vi "Actor Core.vi"(8 "error in":errorcluster, 11 "Progress Window in":refnum<class "Progress Window.lvclass">) -> (0 "error out":errorcluster, 3 "Actor out":refnum<class "Actor.lvclass">)   [LabVIEW 2018, in "Progress Window.lvlib" / "Progress Window.lvclass"]
doc: "(<B>Filename</B>: Actor Framework.lvlib:Actor.lvclass:Actor Core.vi)\n\nReceives messages to the actor, reacts to them, and initiates any error handling that may shut the actor down.\n\nDescendant classes may override this VI to append parallel tasks for the actor to complete while it handles messages. Overrides use the Call Parent Method node."
uses:
  Progress Window.lvclass
  C:/Program Files/National Instruments/LabVIEW 2018/vi.lib/ActorFramework/Actor/Actor.lvclass
  C:/LVCUR/flash-gordon/User Interface/UI Window/UI Window.lvclass
  <vilib>/ActorFramework/Actor/Actor.lvclass
  <vilib>/ActorFramework/Actor/Actor.lvclass/Actor.ctl
  <vilib>/ActorFramework/Message Enqueuer/Message Enqueuer.lvclass/Message Enqueuer.ctl
  <vilib>/ActorFramework/Message Enqueuer/Init from Existing Queue.vi
  <vilib>/ActorFramework/Message Enqueuer/Enqueue.vi
  <vilib>/ActorFramework/Stop Msg/Stop Msg.lvclass
  C:/Program Files/National Instruments/LabVIEW 2018/vi.lib/ActorFramework/Message/Message.lvclass
  Resources/GLOBAL/GLOBAL Time-critical.vi
  <vilib>/ActorFramework/Message Priority Queue/Priority Enqueue.vi
  UI Window/UI Window.lvclass
  <vilib>/ActorFramework/Message Enqueuer/Message Enqueuer.lvclass
panel:
  in  "Stop Button":bool
  out "Recording Movie":u8(slide) scale=0.0..100.0
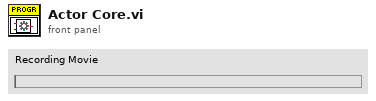
[diagram p1: front panel]
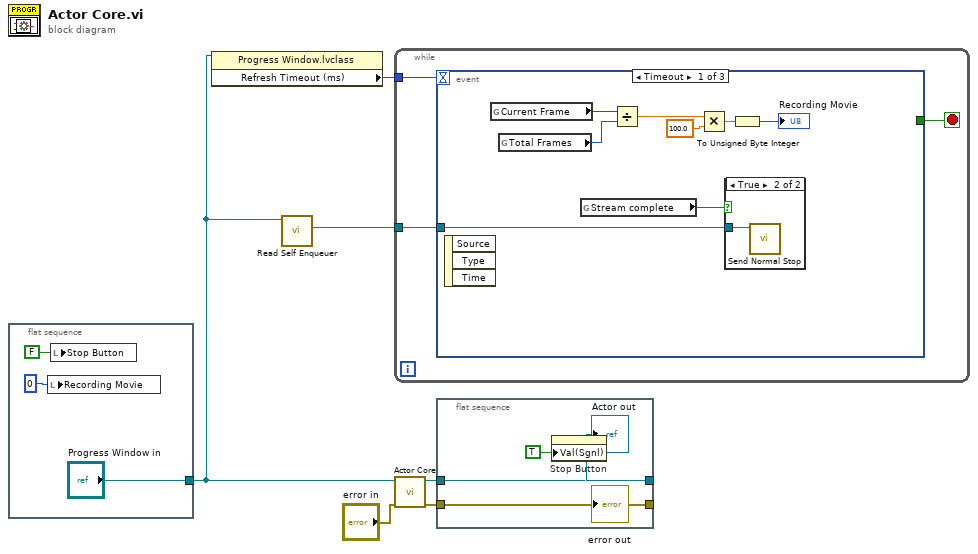
[diagram p0: block diagram]
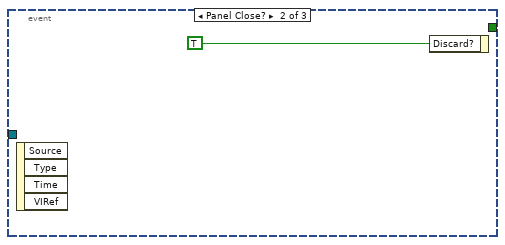
[diagram p3: hidden frame]
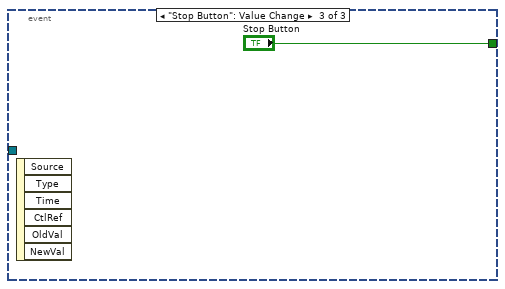
[diagram p4: hidden frame]
diagram:
  n1 = flat-sequence {
    tunnel: ["Progress Window in"] -> w2
    frame #0 {
      n2 = local write "Recording Movie"(u8 0 ("Recording Movie")) -> ()
      n3 = local write "Stop Button"(FALSE ("Stop Button")) -> ()
    }
  }
  n4 = property class="Progress Window.lvclass"(reference=w2) -> ("Refresh Timeout (ms)"=w7:i32)  [unwired: 1 in, 2 out]
  n5 = call <vilib>:"Read Self Enqueuer.vi"("Actor"=w2) -> ("Self Enqueuer"=w1:refnum<class "Message Enqueuer.lvclass">)  [unwired: 10 in]
  n6 = while {
    tunnel: w7 -> [w13]
    tunnel: w1 -> [w14]
    stop <- w12 stop-if-true
    n7 = event shown="[0] Timeout" {
      selector: _ -> [_ _ _]
      dyn-events: _ -> [_ _ _]
      timeout: w13 -> [_ _ _]
      tunnel: w14 -> [w18 _ _]
      tunnel: [_ _ "Stop Button"] -> w12
      event Timeout {
        n8 = event-data() -> ()  [unwired: 1 in, 3 out]
        n9 = global read "GLOBAL Time-critical.vi" "Current Frame"() -> (w17:i32)
        n10 = global read "GLOBAL Time-critical.vi" "Total Frames"() -> (w16:i32)
        n11 = global read "GLOBAL Time-critical.vi" "Stream complete"() -> (w15:bool)
        n12 = Divide(x=w17, y=w16) -> (x/y=w19:dbl)
        n13 = Multiply(x=w19, y=100.0) -> (x*y=w21:dbl)
        n14 = case shown="True" w15 {
          tunnel: w18 -> [_ w23]
          frame False {
          }
          frame True {
            n15 = call <vilib>:"Send Normal Stop.vi"("Message Enqueuer"=w23) -> ()  [unwired: 10 in, 1 out]
          }
        }
        n16 = To Unsigned Byte Integer(number=w21) -> (unsigned 8bit integer=→"Recording Movie":u8)
      }
      event Panel Close? {
        n17 = event-data() -> ()  [unwired: 1 in, 4 out]
        n18 = event-data("Discard?"=TRUE) -> ()  [unwired: 1 in, 1 out]
      }
      event "Stop Button": Value Change {
        n19 = event-data() -> ()  [unwired: 1 in, 6 out]
      }
    }
  }
  n20 = call-parent "Actor Core.vi"("error in"="error in", "UI Window in"=w2) -> ("error out"=w6:errorcluster, "Actor out"=w4:refnum<class "Actor.lvclass">)  [unwired: 8 in]
  n21 = flat-sequence {
    tunnel: w6 -> [w28]
    tunnel: [w28] -> w5
    tunnel: w4 -> [w27]
    tunnel: [w27] -> w3
    frame #0 {
      n22 = property on="Stop Button" class="Bool (strict)"("Val(Sgnl)"=TRUE ("Stop Button")) -> ()  [unwired: 2 in, 2 out]
    }
  }
  "error out" <- w5
  "Actor out" <- w3
